vi "Abort All.vi"(8 "error in (no error)":errorcluster, 11 "Sequencing in":refnum<class "Sequencing.lvclass">) -> (0 "error out":errorcluster, 3 "Sequencing out":refnum<class "Sequencing.lvclass">)   [LabVIEW 2020, in "VolatusSeq.lvlib" / "Sequencing.lvclass"]
uses:
  Sequencing.lvclass
  Sequencing.lvclass/Sequencing.ctl
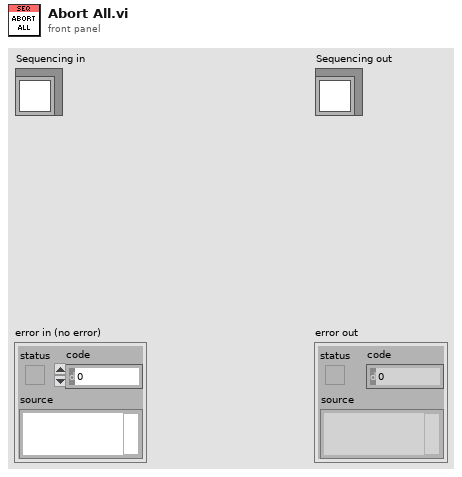
[diagram p1: front panel]
types:
  T1 = typedef "VolatusSeq.lvlib/Sequence Status.ctl" = cluster{"Name":string, "State":string, "Time":T2, "Running":bool, "Start Time":dbl, "Previous Duration":i64, "Previous Late":bool}
  T2 = typedef "VolatusSeq.lvlib/Sequence Time.ctl" = cluster{"Abort":bool, "Seq Time":dbl, "State Time":dbl, "Wall Time":dbl}
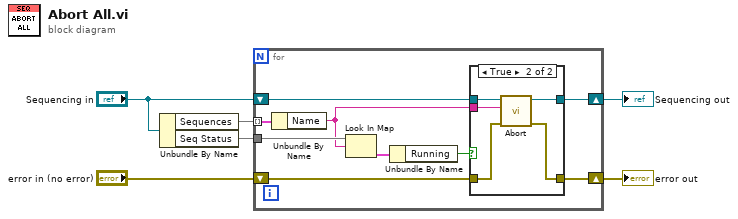
[diagram p0: block diagram]
diagram:
  n1 = Unbundle By Name("Sequencing in") -> ("Sequences"=w6:map{string, refnum<class "Sequence.lvclass">}, "Seq Status"=w4:map{string, T1})
  n2 = for {
    tunnel: w6 -> [w15] mode=indexing
    shift-right: [w8] -> w3
    shift-left: "Sequencing in" -> [w12]
    tunnel: w4 -> [w14]
    shift-right: [w7] -> w1
    shift-left: "error in (no error)" -> [w9]
    n3 = Unbundle By Name(w15) -> ("Name"=w11:string)
    n4 = Look In Map(map=w14, key=w11) -> (value=w13:T1)  [unwired: 1 in, 1 out]
    n5 = Unbundle By Name(w13) -> ("Running"=w10:bool)
    n6 = case shown="True" w10 {
      tunnel: w12 -> [w17 w22]
      tunnel: w11 -> [_ w21]
      tunnel: w9 -> [w16 w20]
      tunnel: [w17 w19] -> w8
      tunnel: [w16 w18] -> w7
      frame False {
      }
      frame True {
        n7 = call "Abort.vi"("error in (no error)"=w20, "Sequence Name"=w21, "Sequencing in"=w22) -> ("error out"=w18:errorcluster, "Sequencing out"=w19:refnum<class "Sequencing.lvclass">)  [unwired: 7 in]
      }
    }
  }
  "error out" <- w1
  "Sequencing out" <- w3
